vi "createDAQmx.vi"(8 "error in (no error)":errorcluster, 10 "DAQ.Config":T1={"Channels"="PXI1Slot2/ao0", "DAQ_Type"=enum."AO", "minimum value"=-5.0, "maximum value"=5.0, "DAQ_SamplingInfo"={"Fs"=1000.0, "#s"=1000}, "DAQ_SamplingMode"=enum."Continuous"} {"maximum value" format="%0.2f"; "minimum value" format="%0.2f"}, 11 "DAQmx in":refnum<class "DAQmx.lvclass">) -> (0 "error out":errorcluster, 3 "DAQmx out":refnum<class "DAQmx.lvclass">)   [LabVIEW 2019, in "DAQmx.lvclass"]
uses:
  DAQmx.lvclass
  DAQ/DAQ.lvclass
  DAQ/Typedefs/DAQ_SamplingMode.ctl
  DAQ/Typedefs/DAQ_SamplingInfo.ctl
  DAQ/Typedefs/PrivateEvents--DAQ.AI.Channels.ctl
  DAQ/Typedefs/DAQ_Type.ctl
  DAQ/Typedefs/DAQ_Config.ctl
panel:
  # "Specific DAQmx config\nWire it to the connector pane"
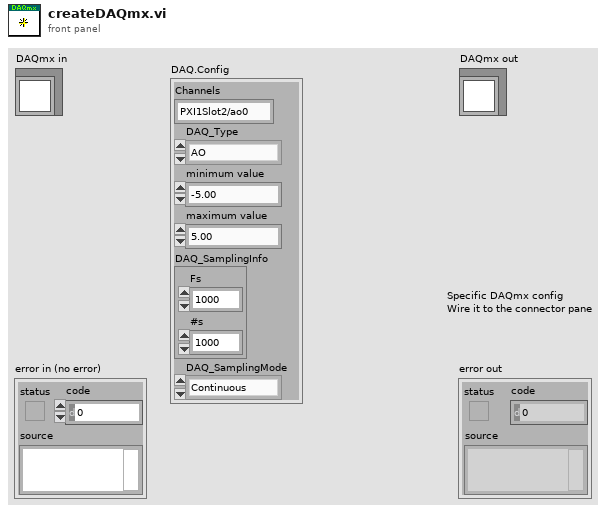
[diagram p1: front panel]
types:
  T1 = typedef "DAQ.lvclass/DAQ_Config.ctl" = cluster{"Channels":T2, "DAQ_Type":T3, "minimum value":dbl, "maximum value":dbl, "DAQ_SamplingInfo":T4, "DAQ_SamplingMode":T5}
  T2 = typedef "DAQ.lvclass/PrivateEvents--DAQ.AI.Channels.ctl" = string
  T3 = typedef "DAQ.lvclass/DAQ_Type.ctl" = enum16{"AI", "AO"}
  T4 = typedef "DAQ.lvclass/DAQ_SamplingInfo.ctl" = cluster{"Fs":dbl, "#s":i32}
  T5 = typedef "DAQ.lvclass/DAQ_SamplingMode.ctl" = enum16{"Continuous", "Finite"}
  T6 = typedef "DAQmx.lvclass/DAQmx_Config.ctl" = cluster{"Buffer Size (S)":i32, "Master Slave":enum16{"MASTER", "SLAVE"}}
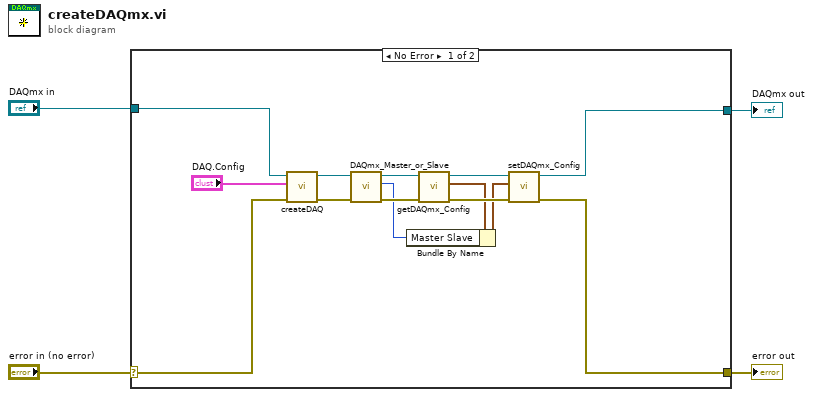
[diagram p0: block diagram]
diagram:
  n1 = case shown="No Error" "error in (no error)" {
    selector: "error in (no error)" -> [w15 w20]
    tunnel: [w6 w20] -> w3
    tunnel: [w7 w19] -> w1
    tunnel: "DAQmx in" -> [w5 w19]
    frame No Error {
      n2 = call "createDAQ.vi"("error in (no error)"=w15, "DAQ.Config"="DAQ.Config", "DAQ in"=w5) -> ("error out"=w16:errorcluster, "DAQ out"=w17:refnum<class "DAQmx.lvclass">)  [unwired: 7 in]
      n3 = call "DAQmx_Master_or_Slave.vi"("error in (no error)"=w16, "DAQmx in"=w17) -> ("error out"=w14:errorcluster, "Enum"=w8:enum16{"MASTER", "SLAVE"}, "DAQmx out"=w13:refnum<class "DAQmx.lvclass">)  [unwired: 7 in]
      n4 = call "getDAQmx_Config.vi"("error in (no error)"=w14, "DAQmx in"=w13) -> ("error out"=w11:errorcluster, "DAQmx.Config"=w10:T6, "DAQmx out"=w12:refnum<class "DAQmx.lvclass">)  [unwired: 7 in]
      n5 = Bundle By Name(cluster=w10, "Master Slave"=w8) -> (w9:T6)
      n6 = call "setDAQmx_Config.vi"("error in (no error)"=w11, "DAQmx.Config"=w9, "DAQmx in"=w12) -> ("error out"=w6:errorcluster, "DAQmx out"=w7:refnum<class "DAQmx.lvclass">)  [unwired: 7 in]
    }
    frame Error {
    }
  }
  "error out" <- w3
  "DAQmx out" <- w1
